vi "Analysis.Calc SPC from 1D Float.vi"(10 "Values":dbl[](array[numeric]), 11 "Limits":T1) -> (3 "SPC Data":string[](array[string]))   [LabVIEW 2024]
uses:
  Analysis.Measurement Limit Info.ctl
  <vilib>/Analysis/NI_AALBase.lvlib
panel:
  # "Name, LL, UL, Min, Max, Mean, Stdev, Cpk"
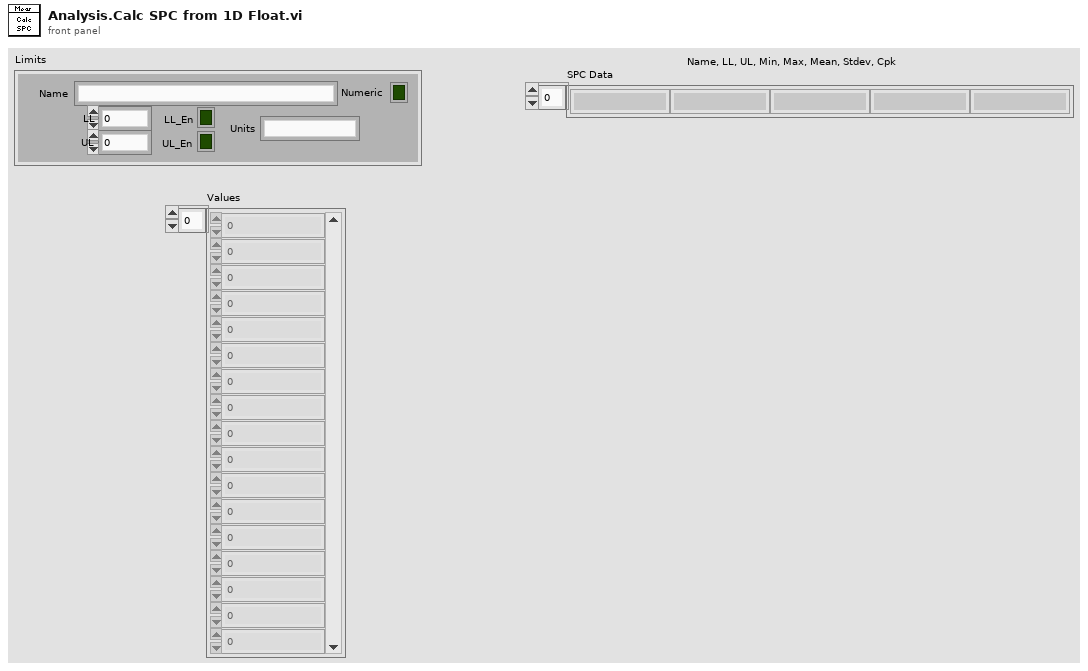
[diagram p1: front panel]
types:
  T1 = typedef "Analysis.Measurement Limit Info.ctl" = cluster{"Name":string, "Numeric":bool, "LL":dbl, "LL_En":bool, "UL":dbl, "UL_En":bool, "Units":string}
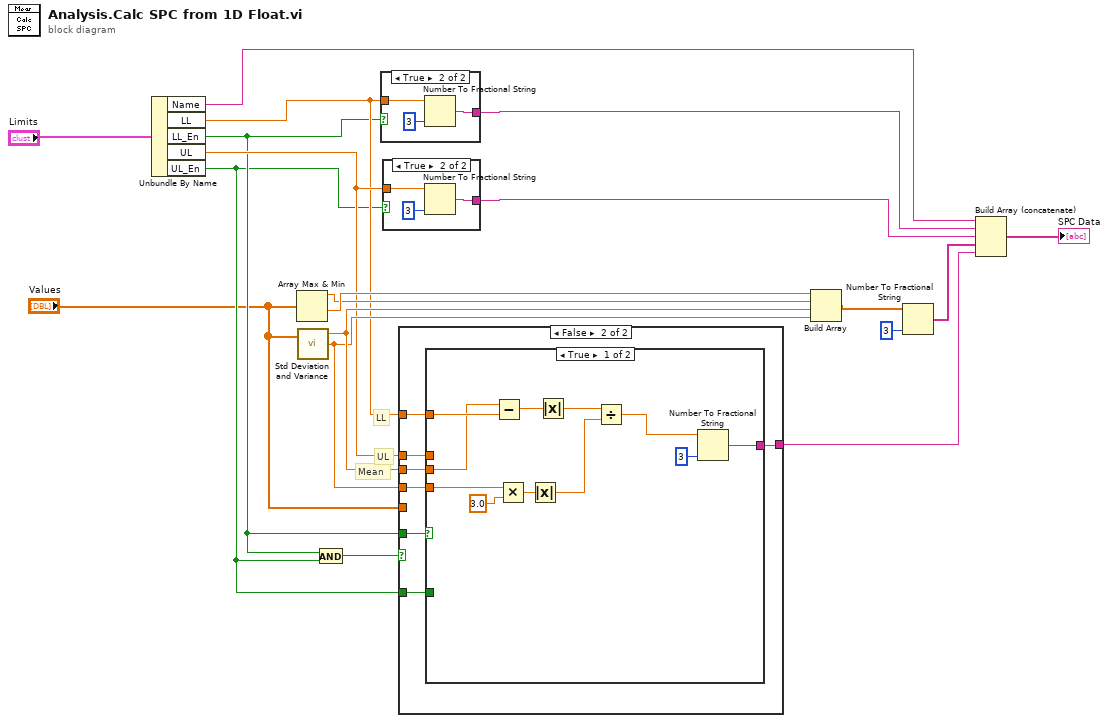
[diagram p0: block diagram]
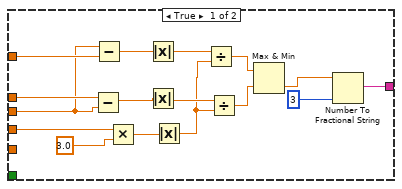
[diagram p2: hidden frame]
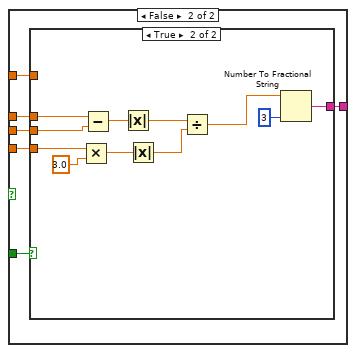
[diagram p3: hidden frame]
diagram:
  # "UL"
  # "LL"
  # "Mean"
  n1 = Unbundle By Name("Limits") -> ("Name"=w16:string, "LL"=w5:dbl, "LL_En"=w4:bool, "UL"=w6:dbl, "UL_En"=w3:bool)
  n2 = Array Max & Min(array="Values") -> (max value=w18:dbl, min value=w19:dbl)  [unwired: 2 out]
  n3 = call <vilib>:"Std Deviation and Variance.vi"("X"="Values") -> ("mean"=w9:dbl, "standard deviation"=w8:dbl)  [unwired: 1 in, 1 out]
  n4 = And(x=w4, y=w3) -> (x .and. y?=w7:bool)
  n5 = case shown="True" w4 {
    tunnel: [_ w22] -> w15
    tunnel: w5 -> [_ w21]
    frame False {
    }
    frame True {
      n6 = Number To Fractional String(number=w21, precision (6)=i16 3) -> (F-format string=w22:string)  [unwired: 2 in]
    }
  }
  n7 = case shown="True" w3 {
    tunnel: [_ w25] -> w14
    tunnel: w6 -> [_ w24]
    frame False {
    }
    frame True {
      n8 = Number To Fractional String(number=w24, precision (6)=i16 3) -> (F-format string=w25:string)  [unwired: 2 in]
    }
  }
  n9 = case shown="False" w7 {
    tunnel: "Values" -> [_ _]
    tunnel: w9 -> [w37 w45]
    tunnel: w8 -> [w41 w48]
    tunnel: w6 -> [w39 w47]
    tunnel: w5 -> [w38 w46]
    tunnel: [w33 w43] -> w2
    tunnel: w4 -> [_ w44]
    tunnel: w3 -> [_ w42]
    frame True {
      n10 = Subtract(x=w39, y=w37) -> (x-y=w30:dbl)
      n11 = Subtract(x=w37, y=w38) -> (x-y=w31:dbl)
      n12 = Multiply(x=w41, y=3.0) -> (x*y=w27:dbl)
      n13 = Absolute Value(x=w31) -> (abs(x)=w28:dbl)
      n14 = Absolute Value(x=w30) -> (abs(x)=w29:dbl)
      n15 = Absolute Value(x=w27) -> (abs(x)=w26:dbl)
      n16 = Divide(x=w28, y=w26) -> (x/y=w36:dbl)
      n17 = Divide(x=w29, y=w26) -> (x/y=w35:dbl)
      n18 = Max & Min(x=w36, y=w35) -> (min(x,y)=w32:dbl)  [unwired: 1 out]
      n19 = Number To Fractional String(number=w32, precision (6)=i16 3) -> (F-format string=w33:string)  [unwired: 2 in]
    }
    frame False {
      n20 = case shown="True" w44 {
        tunnel: w48 -> [w59 w65]
        tunnel: w47 -> [_ w64]
        tunnel: w46 -> [w57 w63]
        tunnel: w45 -> [w56 w62]
        tunnel: [w54 w61] -> w43
        tunnel: w42 -> [_ w60]
        frame True {
          n21 = Subtract(x=w56, y=w57) -> (x-y=w52:dbl)
          n22 = Multiply(x=w59, y=3.0) -> (x*y=w50:dbl)
          n23 = Absolute Value(x=w50) -> (abs(x)=w49:dbl)
          n24 = Absolute Value(x=w52) -> (abs(x)=w51:dbl)
          n25 = Divide(x=w51, y=w49) -> (x/y=w53:dbl)
          n26 = Number To Fractional String(number=w53, precision (6)=i16 3) -> (F-format string=w54:string)  [unwired: 2 in]
        }
        frame False {
          n27 = case shown="True" w60 {
            tunnel: w65 -> [_ w76]
            tunnel: w64 -> [_ w74]
            tunnel: w63 -> [_ _]
            tunnel: w62 -> [_ w73]
            tunnel: [_ w71] -> w61
            frame False {
              # "N/A"
            }
            frame True {
              n28 = Multiply(x=w76, y=3.0) -> (x*y=w67:dbl)
              n29 = Subtract(x=w74, y=w73) -> (x-y=w69:dbl)
              n30 = Absolute Value(x=w69) -> (abs(x)=w68:dbl)
              n31 = Absolute Value(x=w67) -> (abs(x)=w66:dbl)
              n32 = Divide(x=w68, y=w66) -> (x/y=w70:dbl)
              n33 = Number To Fractional String(number=w70, precision (6)=i16 3) -> (F-format string=w71:string)  [unwired: 2 in]
            }
          }
        }
      }
    }
  }
  n34 = Build Array(w19, w18, w9, w8) -> (w12:dbl[])
  n35 = Number To Fractional String(number=w12, precision (6)=i16 3) -> (F-format string=w11:string[])  [unwired: 2 in]
  n36 = Build Array (concatenate)(w16, w15, w14, w11, w2) -> (→"SPC Data":string[])
